vi "SortingArea.vi"(5 "Ring Ref":refnum<vi>, 6 "RingQueue Ref":refnum<vi>, 7 "Peg Ref":refnum<vi>, 8 "Current Area Detect":bool, 9 "Prev Area Detect":bool, 10 "Current Metal Detect":bool, 11 "Prev Metal Detect":bool) -> (2 "Sorting Solenoid Out":bool)   [LabVIEW 2016]
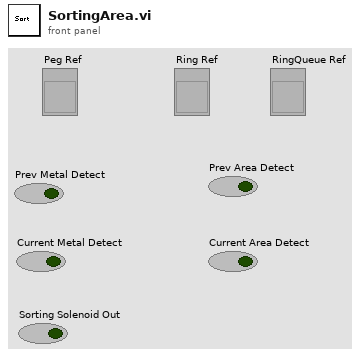
[diagram p1: front panel]
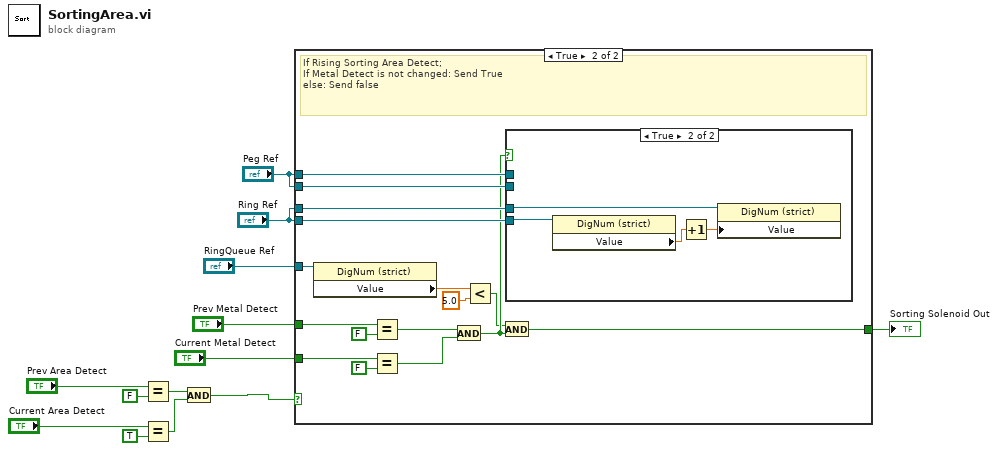
[diagram p0: block diagram]
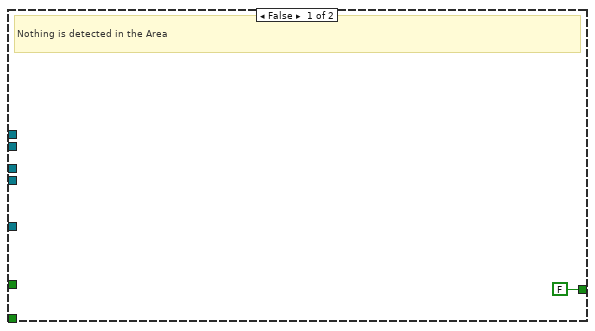
[diagram p2: hidden frame]
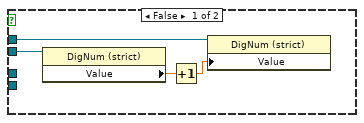
[diagram p3: hidden frame]
diagram:
  n1 = Equal?(x="Prev Area Detect", y=FALSE) -> (x = y?=w3:bool)
  n2 = Equal?(x="Current Area Detect", y=TRUE) -> (x = y?=w2:bool)
  n3 = And(x=w3, y=w2) -> (x .and. y?=w1:bool)
  n4 = case shown="True" w1 {
    tunnel: "Prev Metal Detect" -> [_ w27]
    tunnel: "Current Metal Detect" -> [_ w28]
    tunnel: [FALSE w15] -> w4
    tunnel: "Peg Ref" -> [_ w24]
    tunnel: "Peg Ref" -> [_ w23]
    tunnel: "Ring Ref" -> [_ w22]
    tunnel: "Ring Ref" -> [_ w21]
    tunnel: "RingQueue Ref" -> [_ w20]
    frame False {
      # "Nothing is detected in the Area"
    }
    frame True {
      # "If Rising Sorting Area Detect;\nIf Metal Detect is not changed: Send True\nelse: Send false"
      n5 = property class="DigNum (strict)"(reference=w20) -> ("Value"=w19:dbl)  [unwired: 1 in, 2 out]
      n6 = Equal?(x=w27, y=FALSE) -> (x = y?=w26:bool)
      n7 = Equal?(x=w28, y=FALSE) -> (x = y?=w25:bool)
      n8 = And(x=w26, y=w25) -> (x .and. y?=w17:bool)
      n9 = Less?(x=w19, y=5.0) -> (x < y?=w16:bool)
      n10 = And(x=w16, y=w17) -> (x .and. y?=w15:bool)
      n11 = case shown="True" w17 {
        tunnel: w24 -> [w32 _]
        tunnel: w23 -> [w31 _]
        tunnel: w22 -> [_ w36]
        tunnel: w21 -> [_ w35]
        frame False {
          n12 = property class="DigNum (strict)"(reference=w32) -> ("Value"=w34:dbl)  [unwired: 1 in, 2 out]
          n13 = Increment(x=w34) -> (x+1=w33:dbl)
          n14 = property class="DigNum (strict)"(reference=w31, "Value"=w33) -> ()  [unwired: 1 in, 2 out]
        }
        frame True {
          n15 = property class="DigNum (strict)"(reference=w36) -> ("Value"=w38:dbl)  [unwired: 1 in, 2 out]
          n16 = Increment(x=w38) -> (x+1=w37:dbl)
          n17 = property class="DigNum (strict)"(reference=w35, "Value"=w37) -> ()  [unwired: 1 in, 2 out]
        }
      }
    }
  }
  "Sorting Solenoid Out" <- w4
